vi "Range to mA Span.vi"(5 "Span":T1={"mA Range (0 : 0-20mA)"=0, "Enable Span (False)"=FALSE, "Lower Span (0.000)"=0.0, "Upper Span (20.000)"=20.0, "Bias (0)"=0.0} {"mA Range (0 : 0-20mA)" items=["0-20mA"]; "Upper Span (20.000)" min=-99999.0 max=99999.0 step=1.0 format="%_5g"; "Lower Span (0.000)" min=-99999.0 max=99999.0 step=1.0 format="%_5g"}, 7 "Scaling? (False)":bool, 9 "Floating Point Position (2)":i32=2) -> (6 "Lower Span":i32=-2000 min=-99999 max=99999 step=1, 8 "Upper Span":i32=2000 min=-99999 max=99999 step=1, 10 "Bias":i32)   [LabVIEW 2020, in "Yokogawa GX Series.lvlib"]
doc: "This VI gets the voltage span value from the range."
uses:
  <instrlib>/Yokogawa GX Series/Yokogawa GX Series.lvlib
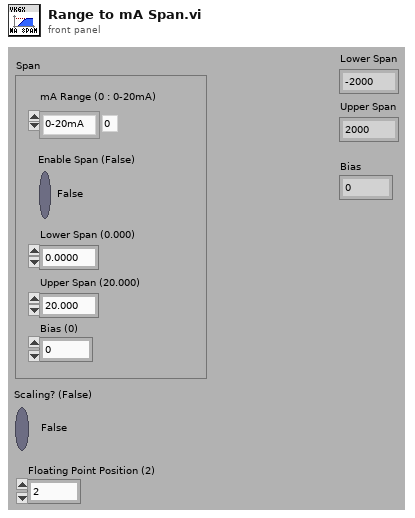
[diagram p1: front panel]
types:
  T1 = cluster{"mA Range (0 : 0-20mA)":i32, "Enable Span (False)":bool, "Lower Span (0.000)":dbl, "Upper Span (20.000)":dbl, "Bias (0)":dbl}
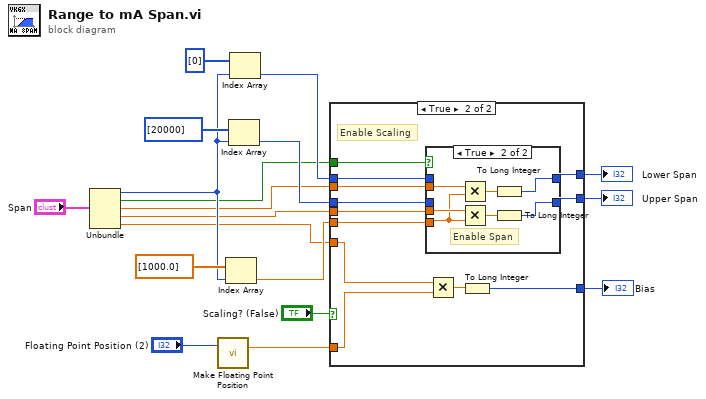
[diagram p0: block diagram]
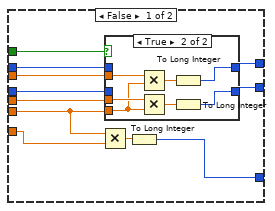
[diagram p2: hidden frame]
diagram:
  n1 = Unbundle("Span") -> ("mA Range (0 : 0-20mA)"=w6:i32, "Enable Span (False)"=w1:bool, "Lower Span (0.000)"=w4:dbl, "Upper Span (20.000)"=w3:dbl, "Bias (0)"=w2:dbl)
  n2 = call <instrlib>:"Make Floating Point Position.vi"("Floating Point Position (2)"="Floating Point Position (2)") -> ("Times"=w13:dbl)  [unwired: 14 in]
  n3 = Index Array(array=dbl[] [1000.0], index=w6) -> (element=w5:dbl)
  n4 = Index Array(array=i32[] [20000], index=w6) -> (element=w8:i32)
  n5 = Index Array(array=i32[] [0], index=w6) -> (element=w10:i32)
  n6 = case shown="True" "Scaling? (False)" {
    tunnel: w5 -> [w21 w42]
    tunnel: w10 -> [w29 w50]
    tunnel: w8 -> [w28 w49]
    tunnel: [w27 w48] -> w18
    tunnel: [w26 w47] -> w17
    tunnel: [w19 w41] -> w16
    tunnel: w2 -> [w20 w40]
    tunnel: w3 -> [w25 w45]
    tunnel: w4 -> [w24 w46]
    tunnel: w1 -> [w23 w44]
    tunnel: w13 -> [_ w39]
    frame False {
      n7 = Multiply(x=w21, y=w20) -> (x*y=w22:dbl)
      n8 = case shown="True" w23 {
        tunnel: w24 -> [_ w37]
        tunnel: w25 -> [_ w36]
        tunnel: [w31 w34] -> w27
        tunnel: [w30 w33] -> w26
        tunnel: w29 -> [w31 _]
        tunnel: w28 -> [w30 _]
        tunnel: w21 -> [_ w32]
        frame False {
        }
        frame True {
          n9 = Multiply(x=w37, y=w32) -> (x*y=w38:dbl)
          n10 = Multiply(x=w36, y=w32) -> (x*y=w35:dbl)
          n11 = To Long Integer(number=w38) -> (32bit integer=w34:i32)
          n12 = To Long Integer(number=w35) -> (32bit integer=w33:i32)
        }
      }
      n13 = To Long Integer(number=w22) -> (32bit integer=w19:i32)
    }
    frame True {
      # "Enable Scaling"
      n14 = case shown="True" w44 {
        tunnel: w46 -> [_ w58]
        tunnel: w45 -> [_ w57]
        tunnel: [w52 w55] -> w48
        tunnel: [w51 w54] -> w47
        tunnel: w50 -> [w52 _]
        tunnel: w49 -> [w51 _]
        tunnel: w42 -> [_ w53]
        frame False {
        }
        frame True {
          # "Enable Span"
          n15 = Multiply(x=w58, y=w53) -> (x*y=w59:dbl)
          n16 = Multiply(x=w57, y=w53) -> (x*y=w56:dbl)
          n17 = To Long Integer(number=w59) -> (32bit integer=w55:i32)
          n18 = To Long Integer(number=w56) -> (32bit integer=w54:i32)
        }
      }
      n19 = Multiply(x=w40, y=w39) -> (x*y=w43:dbl)
      n20 = To Long Integer(number=w43) -> (32bit integer=w41:i32)
    }
  }
  "Lower Span" <- w18
  "Upper Span" <- w17
  "Bias" <- w16
